vi "hidden_error.vi"(8 "Weight":dbl[][](array[numeric]), 10 "Output":dbl[](array[numeric]), 11 "Target":dbl[](array[numeric])) -> (1 "Error_out":dbl[](array[numeric]))   [LabVIEW 2016]
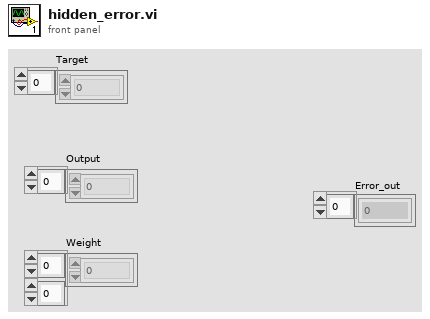
[diagram p1: front panel]
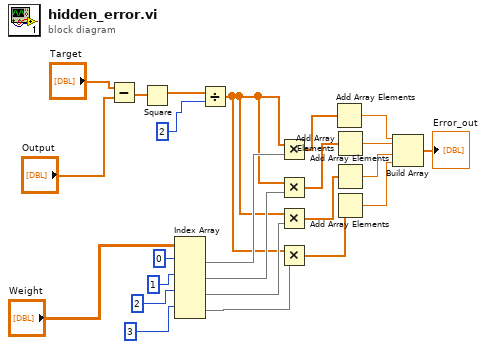
[diagram p0: block diagram]
diagram:
  n1 = Subtract(x="Target", y="Output") -> (x-y=w22:dbl[])
  n2 = Square(x=w22) -> (x^2=w21:dbl[])
  n3 = Index Array(array="Weight", index (row) #1=0 ("index (row)"), index (row) #2=1 ("index (row)"), index (row) #3=2 ("index (row)"), index (row) #4=3 ("index (row)")) -> (element #1=w11:dbl[], element #2=w12:dbl[], element #3=w13:dbl[], element #4=w14:dbl[])  [unwired: 4 in]
  n4 = Divide(x=w21, y=2 ("Numeric")) -> (x/y=w10:dbl[])
  n5 = Multiply(x=w10, y=w11) -> (x*y=w9:dbl[])
  n6 = Multiply(x=w10, y=w12) -> (x*y=w8:dbl[])
  n7 = Multiply(x=w10, y=w13) -> (x*y=w7:dbl[])
  n8 = Multiply(x=w10, y=w14) -> (x*y=w6:dbl[])
  n9 = Add Array Elements(numeric array=w9) -> (sum=w2:dbl)
  n10 = Add Array Elements(numeric array=w8) -> (sum=w3:dbl)
  n11 = Add Array Elements(numeric array=w7) -> (sum=w4:dbl)
  n12 = Add Array Elements(numeric array=w6) -> (sum=w5:dbl)
  n13 = Build Array(w2, w3, w4, w5) -> (→"Error_out":dbl[])
